vi "connect_to_target.vi"(8 "error in":errorcluster, 10 "w5500_port":u16, 11 "ip_addr":string) -> (0 "error out":errorcluster, 3 "TCP Network Connection out":refnum<k5>)   [LabVIEW 2021]
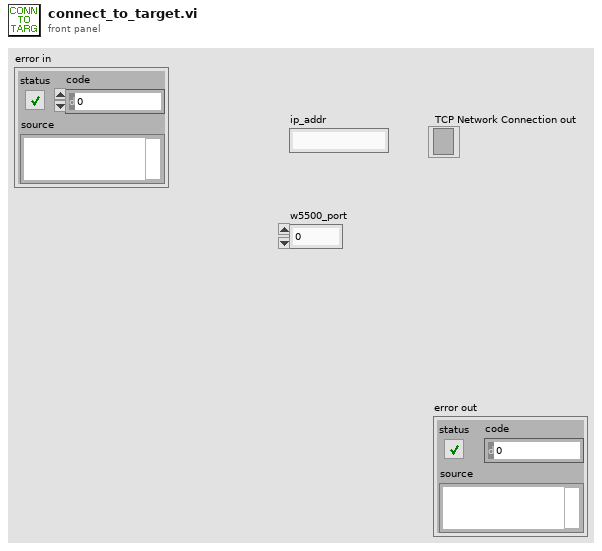
[diagram p1: front panel]
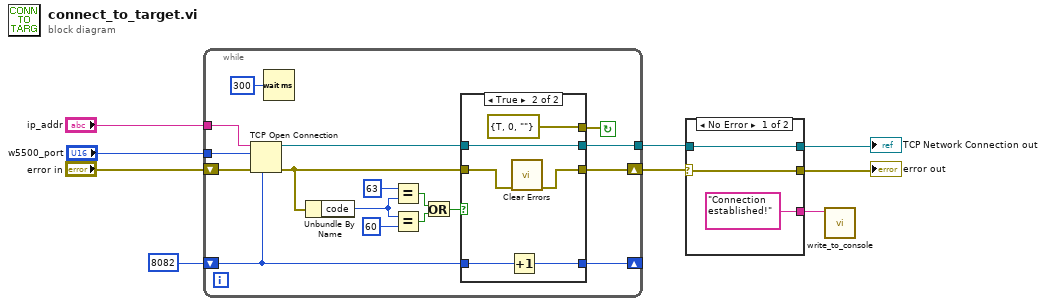
[diagram p0: block diagram]
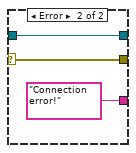
[diagram p2: hidden frame]
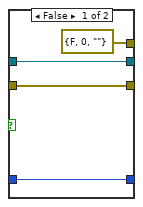
[diagram p3: hidden frame]
diagram:
  n1 = while {
    tunnel: "ip_addr" -> [w26]
    tunnel: "w5500_port" -> [w25]
    tunnel: [w17] -> w5
    shift-right: [w20] -> w4
    shift-left: "error in" -> [w24]
    shift-right: [w19] -> _
    shift-left: u16 8082 ("local port (0)") -> [w21]
    stop <- w15 continue-if-true
    n2 = TCP Open Connection(address=w26, remote port or service name=w25, local port=w21, error in (no error)=w24) -> (connection ID=w18:refnum<k5>, error out=w16:errorcluster)  [unwired: 1 in]
    n3 = Wait (ms)(milliseconds to wait=u32 300) -> ()  [unwired: 1 out]
    n4 = Unbundle By Name(w16) -> ("code"=w14:i32)
    n5 = Equal?(x=63, y=w14) -> (x = y?=w11:bool)
    n6 = Equal?(x=w14, y=60) -> (x = y?=w12:bool)
    n7 = Or(x=w11, y=w12) -> (x .or. y?=w10:bool)
    n8 = case shown="True" w10 {
      tunnel: w21 -> [w30 w34]
      tunnel: w16 -> [w29 w36]
      tunnel: [w29 w35] -> w20
      tunnel: [w30 w33] -> w19
      tunnel: w18 -> [w28 w32]
      tunnel: [w28 w32] -> w17
      tunnel: [errorcluster {"status"=FALSE, "code"=0, "source"=""} ("error IO") errorcluster {"status"=TRUE, "code"=0, "source"=""} ("error IO")] -> w15
      frame False {
      }
      frame True {
        n9 = Increment(x=w34) -> (x+1=w33:u16)
        n10 = call <vilib>:"Clear Errors.vi"("error in (no error)"=w36) -> ("error out"=w35:errorcluster)  [unwired: 5 in, 1 out]
      }
    }
  }
  n11 = case shown="No Error" w4 {
    selector: w4 -> [w37 w40]
    tunnel: w5 -> [w39 w41]
    tunnel: [w39 w41] -> w2
    tunnel: ["Connection established!" "Connection error!"] -> w6
    tunnel: [w37 w40] -> w3
    frame No Error {
    }
    frame Error {
    }
  }
  "TCP Network Connection out" <- w2
  "error out" <- w3
  n12 = call "write_to_console.vi"("input_str"=w6) -> ()  [unwired: 10 in, 1 out]
